vi "Jaguar Control Mode.vi"() -> ()   [LabVIEW 2012]
uses:
  Controls/Jaguar Control Modes.ctl
panel:
  in  "Mode":T1
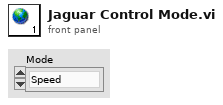
[diagram p1: front panel]
types:
  T1 = typedef "Jaguar Control Modes.ctl" = enum16{"Speed", "Position"}
diagram:
